vi "Analysator Seriennummer setzen.vi"(8 "error in (no error)":errorcluster caption="Fehler (Eingang, kein Fehler)", 10 "Analysator":T1, 11 "String (Eingang)":refnum<vi>) -> (0 "error out":errorcluster caption="Fehler (Ausgang)")   [LabVIEW 2020, in "System Einstellungen V2.lvlib"]
uses:
  System Einstellungen V2.lvlib
  Analysatoren.ctl
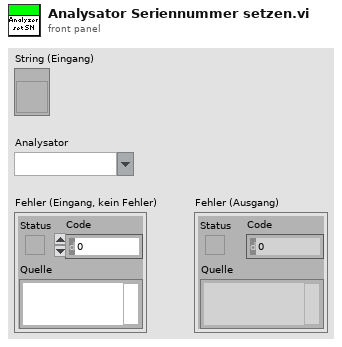
[diagram p1: front panel]
types:
  T1 = typedef "System Einstellungen V2.lvlib/Analysatoren.ctl" = string
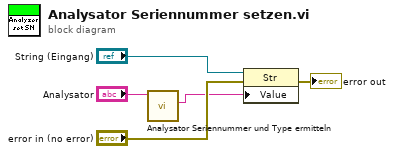
[diagram p0: block diagram]
diagram:
  n1 = call "Analysator Seriennummer und Type ermitteln.vi"("Analysator"="Analysator") -> ("Seriennummer"=w1:string)  [unwired: 8 in, 2 out]
  n2 = property class="Str"(reference="String (Eingang)", error in="error in (no error)", "Value"=w1) -> (error out=→"error out":errorcluster)  [unwired: 1 out]
